vi "Main.vi"   [LabVIEW 2021]
uses:
  Ex Queue Actor/Ex Queue Actor/Ex Queue Actor.lvclass
  C:/git/jettl/src/Actor/Actor/Actor.lvclass
  jettl/jettl Queue Actor/jettl Queue Actor.lvlib
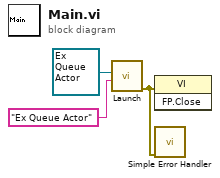
[diagram p0: block diagram]
diagram:
  n1 = call "Launch.vi"("Alias"="Ex Queue Actor", "Actor"=refnum<class "Ex Queue Actor.lvclass"> refnum ("Dev Actor.lvlib:Dev Actor.lvclass")) -> ("error out"=w1:errorcluster)  [unwired: 9 in]
  n2 = invoke class="VI" method="FP.Close"(error in=w1) -> ()  [unwired: 2 in, 3 out]
  n3 = call <vilib>:"Simple Error Handler.vi"("error in (no error)"=w1) -> ()  [unwired: 4 in, 5 out]
